vi "Read Dev.Chassis.vi"(8 "error in (no error)":errorcluster, 11 "SLSC Local in":refnum<class "SLSC Local.lvclass">) -> (0 "error out":errorcluster, 2 "Dev.Chassis":refnum<k21>, 3 "SLSC Local out":refnum<class "SLSC Local.lvclass">)   [LabVIEW 2015, in "SLSC Interfaces.lvlib" / "SLSC Local.lvclass"]
uses:
  SLSC Local.lvclass
  <resource>/objmgr/slsc.rc
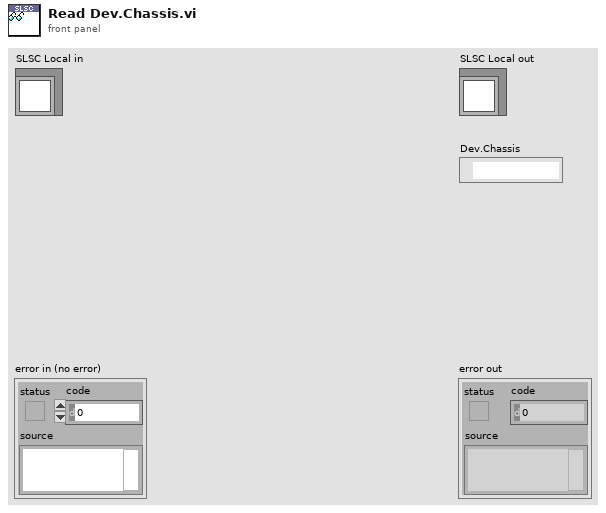
[diagram p1: front panel]
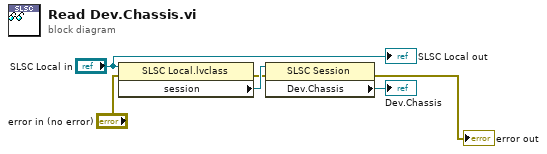
[diagram p0: block diagram]
diagram:
  n1 = property class="SLSC Local.lvclass"(reference="SLSC Local in", error in="error in (no error)") -> (error out=w5:errorcluster, "session"=w6:refnum<k21>)  [unwired: 1 out]
  n2 = property class="SLSC Session"(reference=w6, error in=w5) -> (error out=→"error out":errorcluster, "Dev.Chassis"=→"Dev.Chassis":refnum<k21>)  [unwired: 1 out]
  "SLSC Local out" <- "SLSC Local in"
